vi "split formula.vi"(11 "Formula":string) -> (2 "Symbol":string[](array[string]), 3 "Element":string[](array[string]))   [LabVIEW 2020]
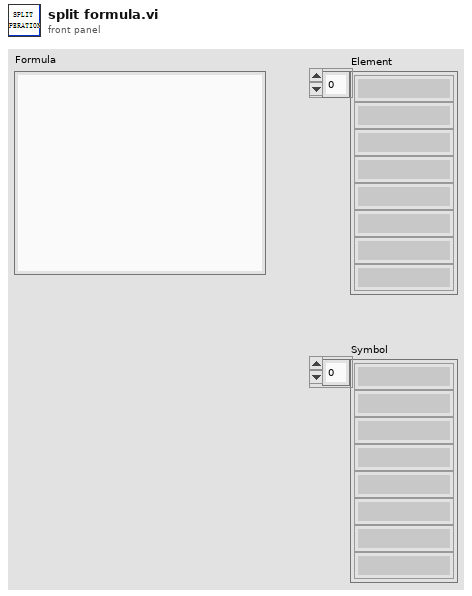
[diagram p1: front panel]
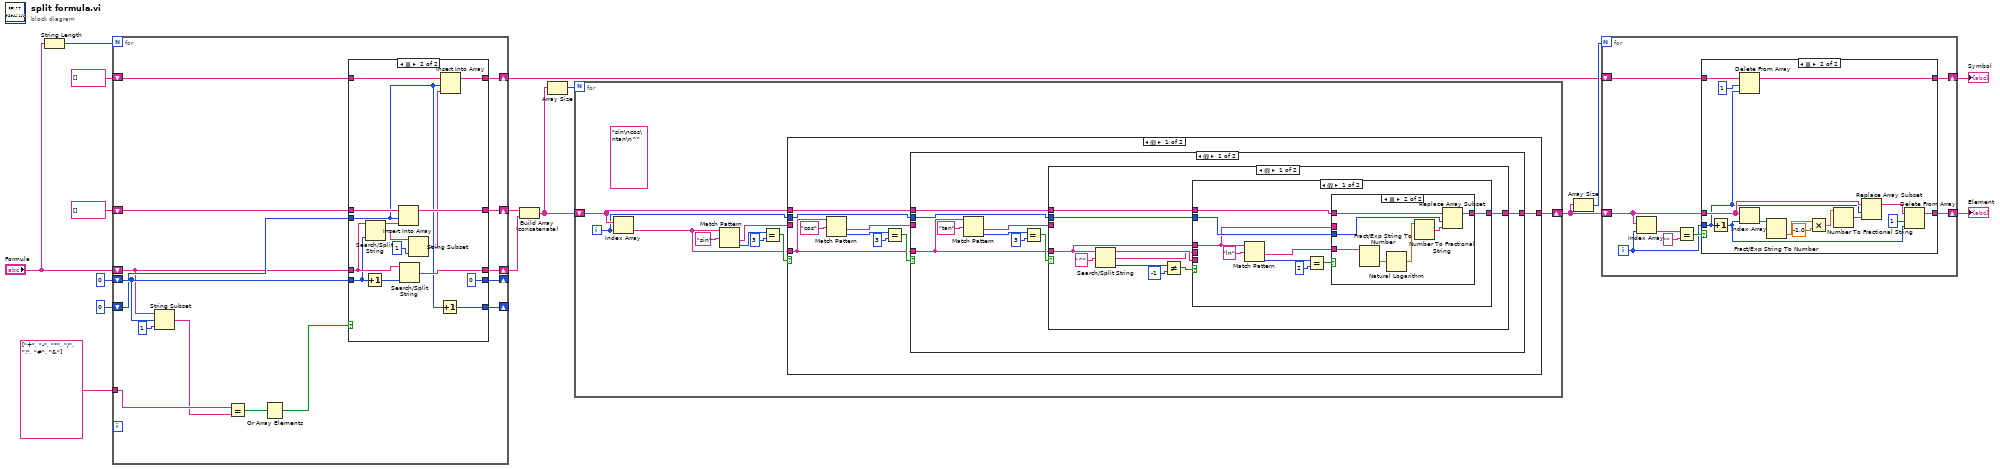
[diagram p0: block diagram]
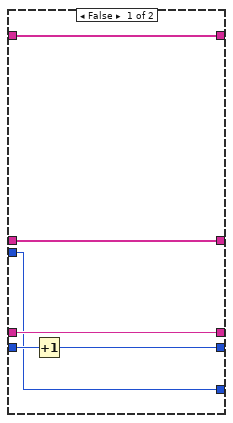
[diagram p3: hidden frame]
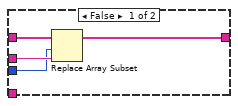
[diagram p4: hidden frame]
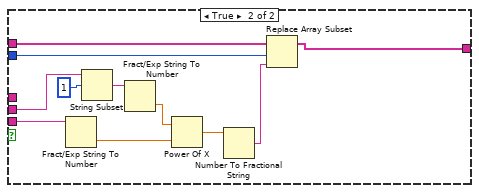
[diagram p5: hidden frame]
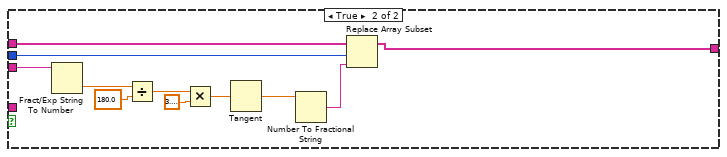
[diagram p6: hidden frame]
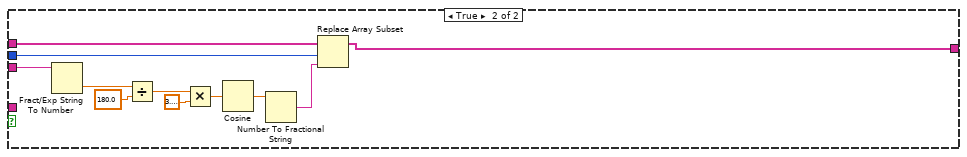
[diagram p7: hidden frame]
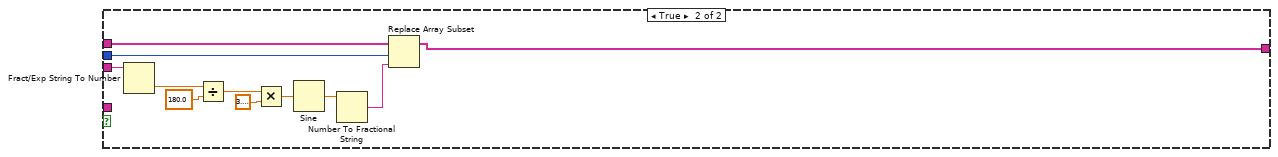
[diagram p8: hidden frame]
diagram:
  n1 = String Length(string="Formula") -> (length=w15:i32)
  n2 = for {
    N: w15 -> [_]
    shift-right: [w22] -> w2
    shift-left: "Formula" -> [w21]
    shift-right: [w29] -> _
    shift-left: 0 -> [w30]
    shift-right: [w28] -> w13
    shift-left: string[] [] -> [w27]
    shift-right: [w25] -> _
    shift-left: 0 -> [w26]
    shift-right: [w23] -> w4
    shift-left: string[] [] -> [w24]
    tunnel: string[] ["+", "-", "*", "/", "!", "#", "&"] -> [w20]
    n3 = String Subset(string=w21, offset (0)=w30, length (rest)=1) -> (substring=w19:string)
    n4 = Equal?(x=w20, y=w19) -> (x = y?=w18:bool[])
    n5 = Or Array Elements(Boolean array=w18) -> (logical OR=w17:bool)
    n6 = case shown="真" w17 {
      tunnel: [w37 w47] -> w22
      tunnel: w21 -> [w37 w49]
      tunnel: w30 -> [w36 w46]
      tunnel: [w35 0] -> w29
      tunnel: [w34 w45] -> w28
      tunnel: w27 -> [w34 w44]
      tunnel: w26 -> [w32 w40]
      tunnel: [w32 w42] -> w25
      tunnel: w24 -> [w33 w41]
      tunnel: [w33 w39] -> w23
      frame False {
        n7 = Increment(x=w36) -> (x+1=w35:i32)
      }
      frame True {
        n8 = Increment(x=w46) -> (x+1=w48:i32)
        n9 = Search/Split String(string=w49, offset (0)=w46) -> (substring before match=w43:string, match + rest of string=w51:string)  [unwired: 1 in, 1 out]
        n10 = Insert Into Array(array=w44, index=w40, new element=w43) -> (w45:string[])
        n11 = Search/Split String(string=w49, offset (0)=w48) -> (match + rest of string=w47:string)  [unwired: 1 in, 2 out]
        n12 = String Subset(string=w51, length (rest)=1 ("长度（剩余）")) -> (substring=w38:string)  [unwired: 1 in]
        n13 = Increment(x=w40) -> (x+1=w42:i32)
        n14 = Insert Into Array(array=w41, index=w40, new element=w38) -> (w39:string[])
      }
    }
  }
  n15 = Build Array (concatenate)(w13, w2) -> (w8:string[])
  n16 = Array Size(array=w8) -> (size(s)=w16:i32)
  n17 = for {
    N: w16 -> [_]
    shift-right: [w53] -> w6
    shift-left: w8 -> [w56]
    i -> [w55]
    (unwired) "sin\ncos\ntan\n^"
    n18 = Index Array(array=w56, index=w55) -> (element=w54:string)
    n19 = Match Pattern(string=w54, regular expression="sin" ("正则表达式")) -> (after substring=w57:string, offset past match=w60:i32)  [unwired: 1 in, 2 out]
    n20 = Equal?(x=w60, y=3) -> (x = y?=w58:bool)
    n21 = case shown="假" w58 {
      tunnel: w57 -> [_ w153]
      tunnel: w56 -> [w65 w146]
      tunnel: w55 -> [w62 w144]
      tunnel: [w64 w143] -> w53
      tunnel: w54 -> [w63 _]
      frame False {
        n22 = Match Pattern(string=w63, regular expression="cos" ("正则表达式")) -> (after substring=w66:string, offset past match=w69:i32)  [unwired: 1 in, 2 out]
        n23 = Equal?(x=w69, y=3) -> (x = y?=w67:bool)
        n24 = case shown="假" w67 {
          tunnel: w66 -> [_ w137]
          tunnel: w65 -> [w74 w134]
          tunnel: [w72 w133] -> w64
          tunnel: w63 -> [w71 _]
          tunnel: w62 -> [w73 w132]
          frame False {
            n25 = Match Pattern(string=w71, regular expression="tan" ("正则表达式")) -> (after substring=w75:string, offset past match=w78:i32)  [unwired: 1 in, 2 out]
            n26 = Equal?(x=w78, y=3) -> (x = y?=w76:bool)
            n27 = case shown="假" w76 {
              tunnel: w75 -> [_ w124]
              tunnel: w74 -> [w82 w123]
              tunnel: w73 -> [w83 w122]
              tunnel: [w81 w121] -> w72
              tunnel: w71 -> [w80 _]
              frame False {
                n28 = Search/Split String(string=w80, search string/char (-)="^" ("搜索字符串/字符(-)")) -> (substring before match=w85:string, match + rest of string=w84:string, offset of match=w88:i32)  [unwired: 1 in]
                n29 = Not Equal?(x=w88, y=-1) -> (x != y?=w86:bool)
                n30 = case shown="假" w86 {
                  tunnel: w85 -> [_ w113]
                  tunnel: w84 -> [_ w120]
                  tunnel: w83 -> [w93 w116]
                  tunnel: w82 -> [w92 w115]
                  tunnel: [w91 w114] -> w81
                  tunnel: w80 -> [w90 _]
                  frame False {
                    n31 = Match Pattern(string=w90, regular expression="ln" ("正则表达式")) -> (after substring=w94:string, offset past match=w97:i32)  [unwired: 1 in, 2 out]
                    n32 = Equal?(x=w97, y=2) -> (x = y?=w95:bool)
                    n33 = case shown="真" w95 {
                      tunnel: w94 -> [_ w109]
                      tunnel: w93 -> [w101 w105]
                      tunnel: w92 -> [w100 w104]
                      tunnel: [w99 w103] -> w91
                      tunnel: w90 -> [w102 _]
                      frame False {
                        n34 = Replace Array Subset(array=w100, new element=w102, index=w101) -> (w99:string[])
                      }
                      frame True {
                        n35 = Fract/Exp String To Number(string=w109) -> (number=w108:dbl)  [unwired: 3 in, 1 out]
                        n36 = Natural Logarithm(1:w108) -> (0:w107:dbl)
                        n37 = Number To Fractional String(number=w107) -> (F-format string=w106:string)  [unwired: 3 in]
                        n38 = Replace Array Subset(array=w104, new element=w106, index=w105) -> (w103:string[])
                      }
                    }
                  }
                  frame True {
                    n39 = Fract/Exp String To Number(string=w113) -> (number=w112:dbl)  [unwired: 3 in, 1 out]
                    n40 = String Subset(string=w120, offset (0)=1 ("偏移量(0)")) -> (substring=w111:string)  [unwired: 1 in]
                    n41 = Fract/Exp String To Number(string=w111) -> (number=w110:dbl)  [unwired: 3 in, 1 out]
                    n42 = Power Of X(1:w112, 2:w110) -> (0:w118:dbl)
                    n43 = Number To Fractional String(number=w118) -> (F-format string=w117:string)  [unwired: 3 in]
                    n44 = Replace Array Subset(array=w115, new element=w117, index=w116) -> (w114:string[])
                  }
                }
              }
              frame True {
                n45 = Fract/Exp String To Number(string=w124) -> (number=w131:dbl)  [unwired: 3 in, 1 out]
                n46 = Divide(x=w131, y=180.0) -> (x/y=w129:dbl)
                n47 = Multiply(x=w129, y=3.141592653589793) -> (x*y=w127:dbl)
                n48 = Tangent(1:w127) -> (0:w126:dbl)
                n49 = Number To Fractional String(number=w126) -> (F-format string=w125:string)  [unwired: 3 in]
                n50 = Replace Array Subset(array=w123, new element=w125, index=w122) -> (w121:string[])
              }
            }
          }
          frame True {
            n51 = Fract/Exp String To Number(string=w137) -> (number=w142:dbl)  [unwired: 3 in, 1 out]
            n52 = Divide(x=w142, y=180.0) -> (x/y=w140:dbl)
            n53 = Multiply(x=w140, y=3.141592653589793) -> (x*y=w136:dbl)
            n54 = Cosine(x=w136) -> (cos(x)=w135:dbl)
            n55 = Number To Fractional String(number=w135) -> (F-format string=w138:string)  [unwired: 3 in]
            n56 = Replace Array Subset(array=w134, new element=w138, index=w132) -> (w133:string[])
          }
        }
      }
      frame True {
        n57 = Fract/Exp String To Number(string=w153) -> (number=w152:dbl)  [unwired: 3 in, 1 out]
        n58 = Divide(x=w152, y=180.0) -> (x/y=w150:dbl)
        n59 = Multiply(x=w150, y=3.141592653589793) -> (x*y=w148:dbl)
        n60 = Sine(x=w148) -> (sin(x)=w147:dbl)
        n61 = Number To Fractional String(number=w147) -> (F-format string=w145:string)  [unwired: 3 in]
        n62 = Replace Array Subset(array=w146, new element=w145, index=w144) -> (w143:string[])
      }
    }
  }
  n63 = Array Size(array=w6) -> (size(s)=w7:i32)
  n64 = for {
    N: w7 -> [_]
    shift-right: [w156] -> w5
    shift-left: w6 -> [w157]
    shift-right: [w154] -> w3
    shift-left: w4 -> [w155]
    i -> [w158]
    n65 = Index Array(array=w157, index=w158) -> (element=w160:string)
    n66 = Equal?(x=w160, y="") -> (x = y?=w161:bool)
    n67 = case shown="真" w161 {
      tunnel: w158 -> [_ w165]
      tunnel: w157 -> [w163 w173]
      tunnel: [w163 w168] -> w156
      tunnel: w155 -> [w162 w167]
      tunnel: [w162 w164] -> w154
      frame False {
      }
      frame True {
        n68 = Increment(x=w165) -> (x+1=w169:i32)
        n69 = Delete From Array(array=w167, length=1 ("长度"), index=w165) -> (array with subset deleted=w164:string[])  [unwired: 1 out]
        n70 = Index Array(array=w173, index=w169) -> (element=w172:string)
        n71 = Fract/Exp String To Number(string=w172) -> (number=w177:dbl)  [unwired: 3 in, 1 out]
        n72 = Multiply(x=w177, y=-1.0) -> (x*y=w175:dbl)
        n73 = Number To Fractional String(number=w175) -> (F-format string=w174:string)  [unwired: 3 in]
        n74 = Replace Array Subset(array=w173, new element=w174, index=w165) -> (w171:string[])
        n75 = Delete From Array(array=w171, length=1 ("长度"), index=w169) -> (array with subset deleted=w168:string[])  [unwired: 1 out]
      }
    }
  }
  "Element" <- w5
  "Symbol" <- w3
